vi "test.vi"() -> ()   [LabVIEW 2014]
uses:
  Stop watch/Stop watch.lvlib
panel:
  in  "stop 4":bool
  in  "check":bool
  out "Elapsed time 4":u32
  out "Timer up 4":bool
  in  "Time to wait, mS 4":dbl format="%#_13g"
  in  "reset timer":bool
  out "Elapsed time 3":u32
  out "Elapsed time 2":u32
  out "Elapsed time":u32
  in  "stop 3":bool
  in  "stop 2":bool
  in  "Time to wait, mS 3":dbl format="%#_13g"
  out "Timer up 3":bool
  in  "Time to wait, mS 2":dbl format="%#_13g"
  out "Timer up 2":bool
  in  "Time to wait, mS":dbl format="%#_13g"
  out "Timer up":bool
  in  "stop":bool
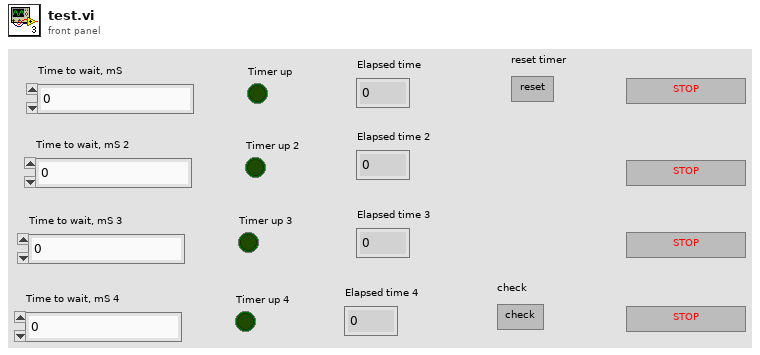
[diagram p1: front panel]
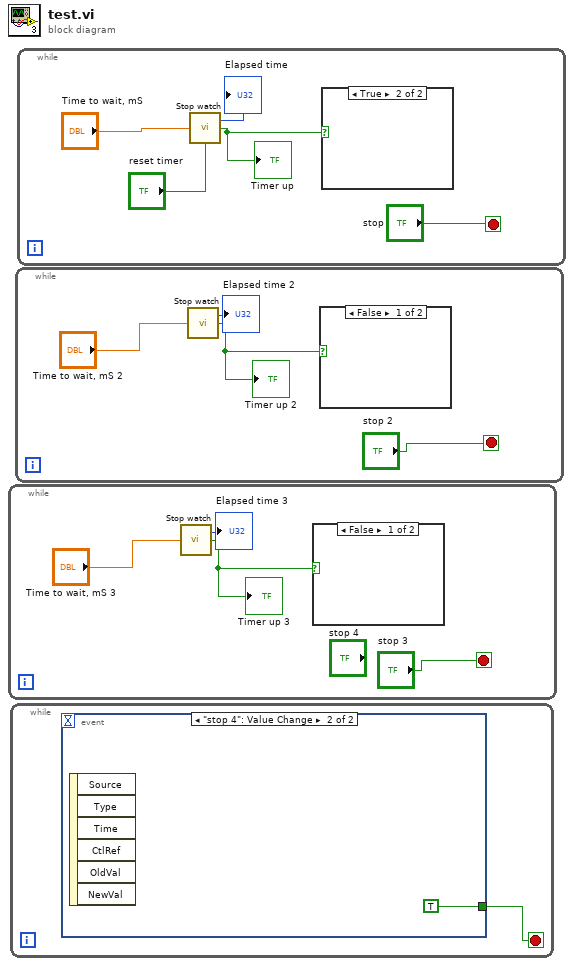
[diagram p0: block diagram]
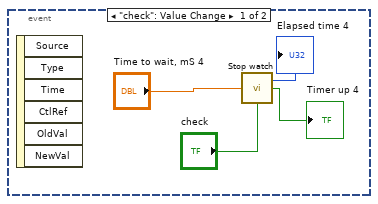
[diagram p2: hidden frame]
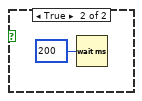
[diagram p3: hidden frame]
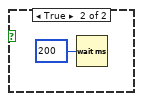
[diagram p4: hidden frame]
diagram:
  n1 = while {
    stop <- "stop 3" stop-if-true
    n2 = call "Stop watch.vi"("Time to wait, mS"="Time to wait, mS 3") -> ("Elapsed time, ms"=→"Elapsed time 3":u32, "Timer up"=w3:bool)  [unwired: 13 in]
    "Timer up 3" <- w3
    n3 = case shown="False" w3 {
      frame False {
      }
      frame True {
        n4 = Wait (ms)(milliseconds to wait=u32 200) -> ()  [unwired: 1 out]
      }
    }
  }
  n5 = while {
    stop <- w6 stop-if-true
    n6 = event shown="[1] \"stop 4\": Value Change" {
      selector: _ -> [_ _]
      dyn-events: _ -> [_ _]
      timeout: _ -> [_ _]
      tunnel: [_ TRUE] -> w6
      event "check": Value Change {
        n7 = event-data() -> ()  [unwired: 1 in, 6 out]
        n8 = call "Stop watch.vi"("Time to wait, mS"="Time to wait, mS 4", "reset timer"="check") -> ("Elapsed time, ms"=→"Elapsed time 4":u32, "Timer up"=→"Timer up 4":bool)  [unwired: 12 in]
      }
      event "stop 4": Value Change {
        n9 = event-data() -> ()  [unwired: 1 in, 6 out]
      }
    }
  }
  n10 = while {
    stop <- "stop 2" stop-if-true
    n11 = call "Stop watch.vi"("Time to wait, mS"="Time to wait, mS 2") -> ("Elapsed time, ms"=→"Elapsed time 2":u32, "Timer up"=w14:bool)  [unwired: 13 in]
    "Timer up 2" <- w14
    n12 = case shown="False" w14 {
      frame False {
      }
      frame True {
        n13 = Wait (ms)(milliseconds to wait=u32 200) -> ()  [unwired: 1 out]
      }
    }
  }
  n14 = while {
    stop <- "stop" stop-if-true
    n15 = call "Stop watch.vi"("Time to wait, mS"="Time to wait, mS", "reset timer"="reset timer") -> ("Elapsed time, ms"=→"Elapsed time":u32, "Timer up"=w20:bool)  [unwired: 12 in]
    "Timer up" <- w20
    n16 = case shown="True" w20 {
      frame False {
      }
      frame True {
      }
    }
  }
